vi "deserialize.vi"(8 "error in":errorcluster, 10 "serialized form":string, 11 "CEF_Configuration in":refnum<class "CEF_serializable configuration.lvclass">) -> (0 "error out":errorcluster, 3 "CEF_Configuration out":refnum<class "CEF_serializable configuration.lvclass">)   [LabVIEW 2023, in "CEF.lvlib" / "CEF_serializable configuration.lvclass"]
doc: "Copyright 2017 National Instruments Corporation\n\nLicensed under the Apache License, Version 2.0 (the \"License\"); you may not use this file except in compliance with the License. You may obtain a copy of the License at http://www.apache.org/licenses/LICENSE-2.0\nUnless required by applicable law or agreed to in writing, software distributed under the License is distributed on an \"AS IS\" BASIS, WITHOUT WARRANTIES OR CONDITIONS OF ANY KIND, either express or implied. See the License for the specific language governing permissions and limitations under the License."
uses:
  CEF_serializable configuration.lvclass
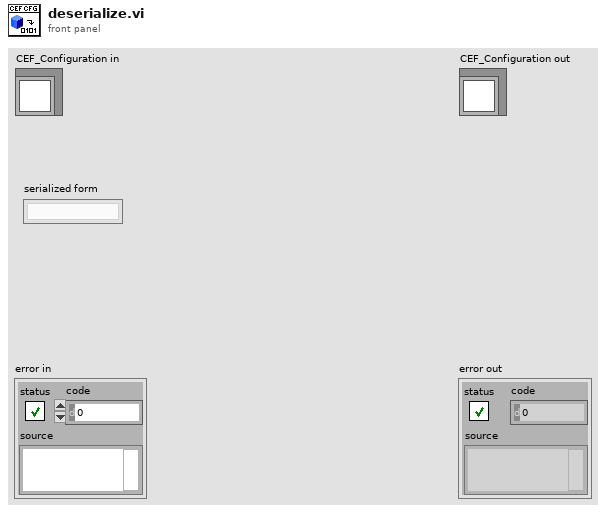
[diagram p1: front panel]
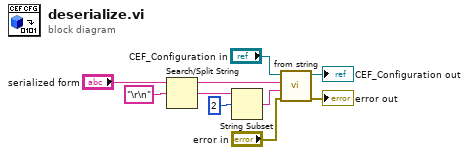
[diagram p0: block diagram]
diagram:
  n1 = Search/Split String(string="serialized form", search string/char (-)="\r\n" ("concatenated string")) -> (substring before match=w1:string, match + rest of string=w4:string)  [unwired: 1 in, 1 out]
  n2 = String Subset(string=w4, offset (0)=2) -> (substring=w2:string)  [unwired: 1 in]
  n3 = call-dynamic "from string.vi"("error in"="error in", "data"=w2, "version"=w1, "CEF_Configuration in"="CEF_Configuration in") -> ("error out"=→"error out":errorcluster, "CEF_Configuration out"=→"CEF_Configuration out":refnum<class "CEF_serializable configuration.lvclass">)  [unwired: 6 in]
